vi "TDOanalysis.vi"() -> ()   [LabVIEW 2018]
uses:
  Libraries/File/Data window.ctl
  <vilib>/Analysis/4window.llb/Hanning Window (DBL).vi
  <vilib>/Analysis/4window.llb/Blackman Window (DBL).vi
  <vilib>/Analysis/baseanly.llb/Mean (DBL).vi
  <vilib>/Analysis/8numeric.llb/1D Numeric Integration.vi
  <vilib>/Analysis/4window.llb/AllCosWindow (DBL).vi
  Libraries/File/File LLB/Read any file Waveform 1ch.vi
  <vilib>/measure/matone.llb/Extract Single Tone Information 1 Chan.vi
  <vilib>/Waveform/WDTOps.llb/WDT Number of Waveform Samples DBL.vi
  <vilib>/Utility/file.llb/Write To Spreadsheet File (DBL).vi
  <vilib>/Analysis/NI_AALPro.lvlib
  <vilib>/measure/NI_MAPro.lvlib
  <vilib>/Analysis/NI_AALBase.lvlib
  <vilib>/Analysis/NI_AAL_SigProc.lvlib
panel:
  in  "Tab Control":T1(tab)
  in  "Input File":path=path "/Users/arkady/Desktop/Dropbox/local_data/rucl3-60T-Oct2018/101118/p003_101118.tdms"
  in  "Power spctr. \nAmpl. threshold":dbl=0.001 format="%.4e"
  in  "Bdot Calibration Factor":dbl=3794.0
  out "TDO Frequency vs. Field":cluster{dbl[], dbl[]}(graph)
  in  "Save Results?":bool=TRUE
  out "B dot offset":dbl=0.00015410527073910347 format="%.6f"
  in  "Data File Type":T2(ring)
  in  "Data channels (1st - Field, 2nd - TDO)":T3={"Start"=0, "Length"=10000, "Other frmt channel numbers"=[0], "TDMS Channel names"=["Field", "Vp"], "TDMS Group name"="p"}
  in  "Length for Bdot offset, s":dbl=0.009 format="%#_6p"
  in  "Input field format":enum16{"Bdot", "B"}(ring)=enum."B"
  in  "Power spctr.\nFreq. threshold":dbl=10000.0
  out "Progress":dbl(slide)=0.9998769230769231 scale=0.0..1.0
  in  "Sliding window width, s":dbl=0.0002 format="%#_6p"
  in  "Sliding window step, s":dbl=2e-05 format="%#_6p"
  in  "Frequency detection md":T4(ring)
  in  "Peak-to-peak  fit width":i32=3 min=3
  in  "Low-pass filter":T5={"Clip IIR filter ramps, in 1/Tc units"=1.0, "Two-pass & flip"=TRUE, "IIR filter specifications"={"Topology"=enum."Off", "Type"=enum."Lowpass", "Order"=1, "Lower Fc"=1e-06, "Upper Fc"=0.0, "PB Ripple"=1.0, "SB Attenuation"=60.0}} {"IIR filter specifications"."PB Ripple" format="%0.2f"; "IIR filter specifications"."Lower Fc" format="%0.2p"; "IIR filter specifications"."SB Attenuation" format="%0.2f"; "IIR filter specifications"."Upper Fc" format="%0.2p"}
  in  "Window type":enum16{"Hanning", "Box", "Blackman"}(ring)
  out "Elapsed time":dbl=1.143
  in  "Field correction":dbl=1.0
  out "Array":bool[](array[boolean])
  out "Background subtracted":cluster{"Output":dbl[], dbl[]}[](graph)
  in  "Background file":path
  out "size(s)":i32=6499
  in  "error in":errorcluster
  in  "lower limit":dbl
  in  "upper limit":dbl
  in  "# of threads":i32=4
  out "Frequency vs. time":waveform(dbl)(graph)={"t0"=timestamp(-0.010000000000000009 s since 1904-01-01), "dt"=2e-05, "Y"=array[6499 elements]}
  out "Field profile":waveform(dbl)(graph)={"t0"=timestamp(-0.010000000000000009 s since 1904-01-01), "dt"=2e-05, "Y"=array[6499 elements]}
  out "TDO Apmlitude or Pwr. vs. Field":cluster{dbl[], dbl[]}(graph)
  out "TDO Amplitude vs. Field (PWR peak)":cluster{dbl[], "Filtered X":dbl[]}(graph)
  in  "End, s":dbl=nan format="%.6f"
  in  "Start, s":dbl=nan format="%.6f"
  in  "Separate file?":bool
  in  "Input Field File (optional)":path
  # "Field  Settings"
  # "TDO Analysis Settings"
  # "Basic NHMFL TDO routine\nv. 0.5       F. F. Balakirev"
  # "OR"
  # "Background file is either an ASCII *.dat file produced by TDO earlier\nor *.fit file containing single column of polynomial fit coeficients.\n1st row in fit file is a text header, which is ingnored. Result is saved in a \n\"*diff.dat\" file in the output folder\nExample \"PDO1.fit\": \n\nFit y=A_i*x^i, starting with A_0\n3.25637E7\n2132.56863\n-12.60591\n-2.01013\n-0.04452\n-3.23119E-4"
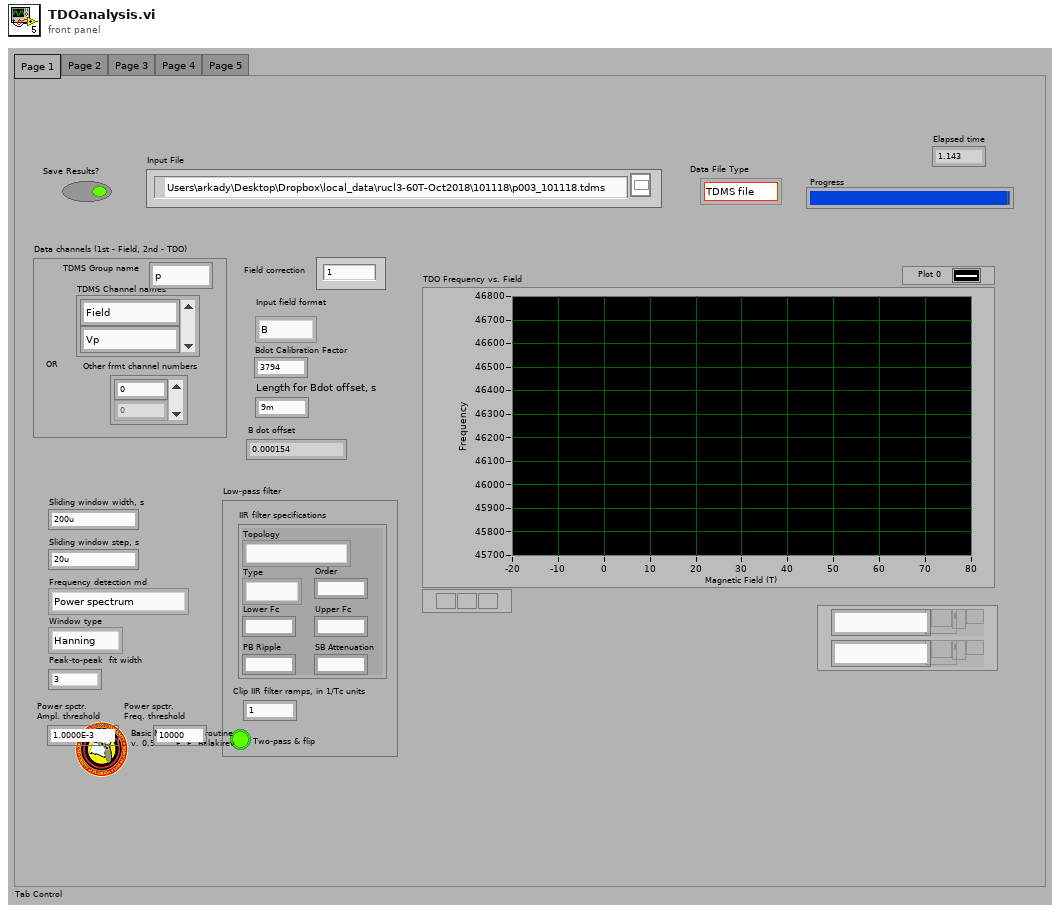
[diagram p1: front panel]
types:
  T1 = enum32{"Page 1", "Page 2", "Page 3", "Page 4", "Page 5"}
  T2 = enum16{"TDMS file", "Tektronics ISF", "BinF file", "ASCII File", "BinH File", "BinW File", "BINARY File"}
  T3 = cluster{"Start":i64, "Length":i32, "Other frmt channel numbers":i64[], "TDMS Channel names":string[], "TDMS Group name":string}
  T4 = enum16{"Power spectrum", "Tone detection", "Peak-to-peak fit"}
  T5 = cluster{"Clip IIR filter ramps, in 1/Tc units":dbl, "Two-pass & flip":bool, "IIR filter specifications":cluster{"Topology":enum16{"Off", "Butterworth", "Chebyshev", "Inverse Chebyshev", "Elliptic", "Bessel"}, "Type":enum16{"Lowpass", "Highpass", "Bandpass", "Bandstop"}, "Order":i32, "Lower Fc":dbl, "Upper Fc":dbl, "PB Ripple":dbl, "SB Attenuation":dbl}}
  T6 = typedef "Data window.ctl" = cluster{"Start":i64, "Length":i64, "Channel numbers":i64[], "Channel name":string, "Group name":string}
  T7 = enum16{"Off", "Butterworth", "Chebyshev", "Inverse Chebyshev", "Elliptic", "Bessel"}
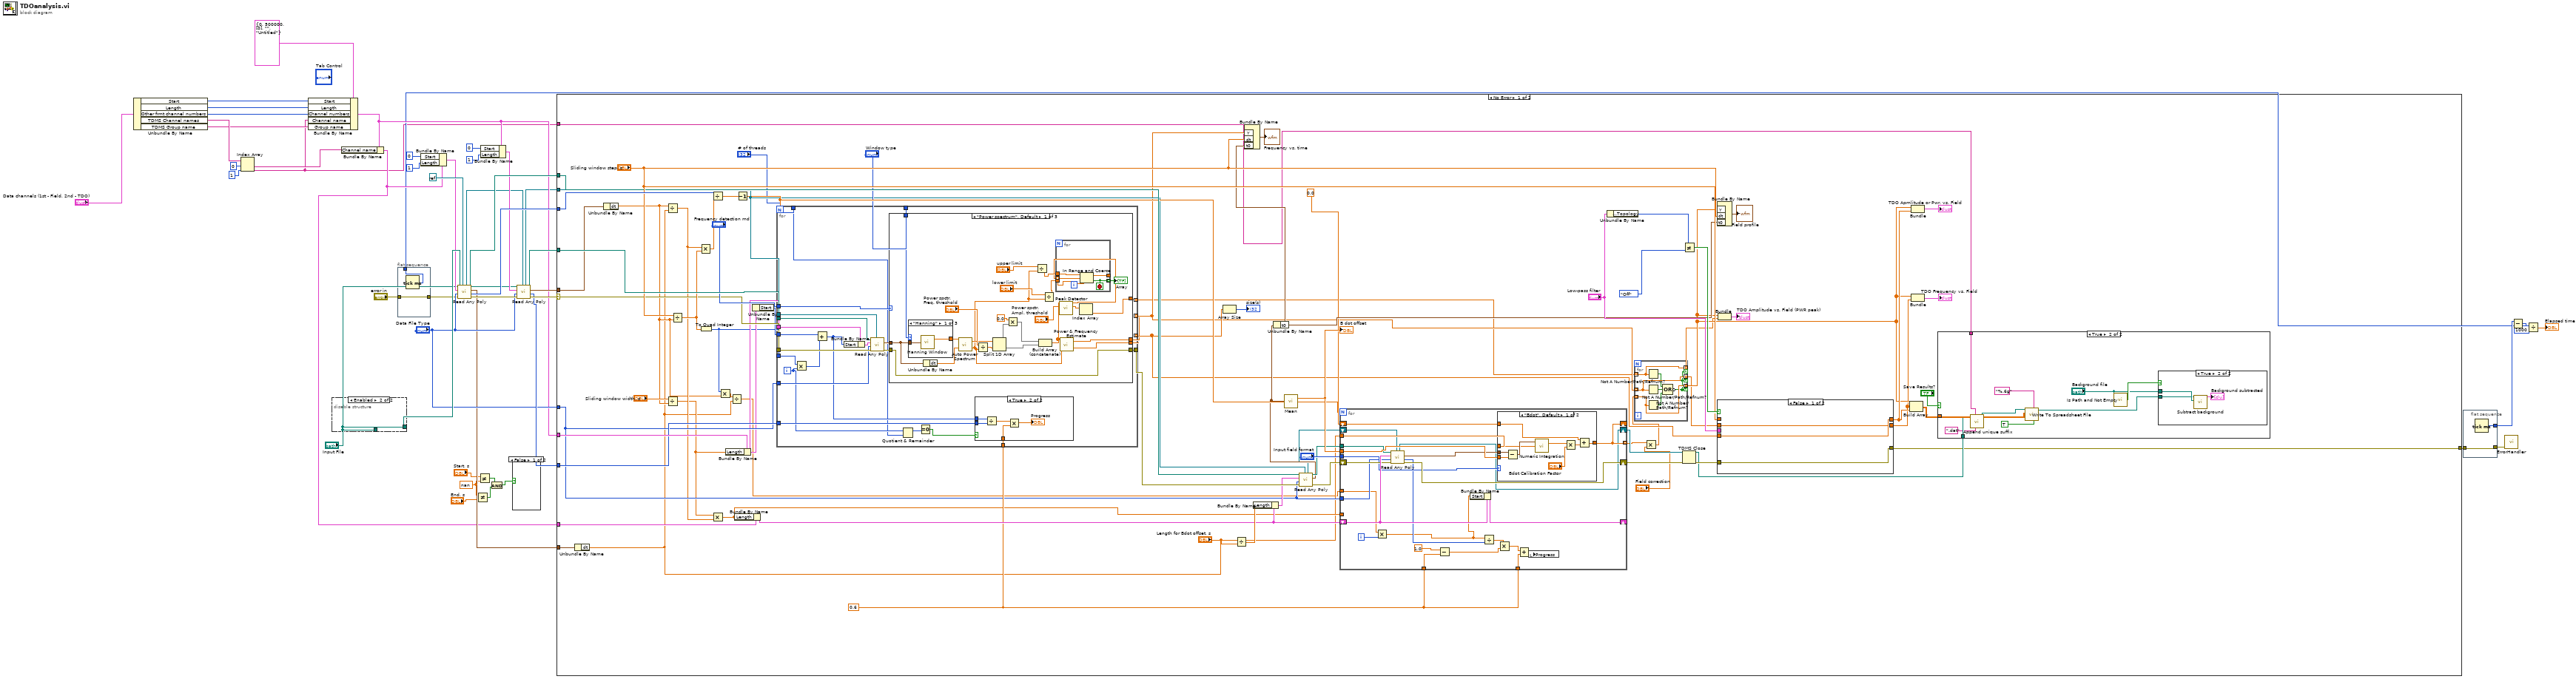
[diagram p0: block diagram]
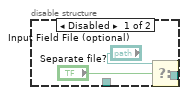
[diagram p2: hidden frame]
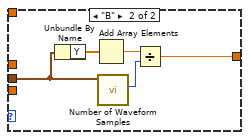
[diagram p4: hidden frame]
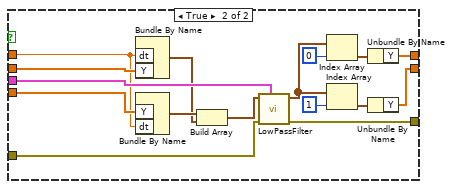
[diagram p5: hidden frame]
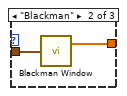
[diagram p9: hidden frame]
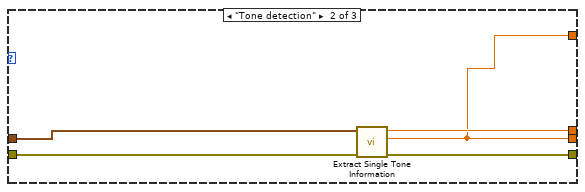
[diagram p11: hidden frame]
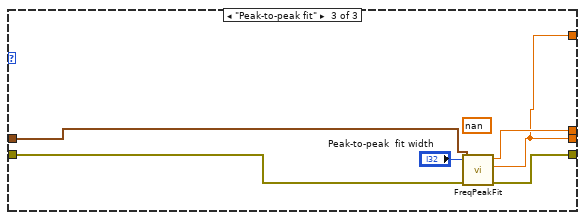
[diagram p12: hidden frame]
diagram:
  w19 = nan
  n1 = Unbundle By Name("Data channels (1st - Field, 2nd - TDO)") -> ("Start"=w30:i64, "Length"=w33:i32, "Other frmt channel numbers"=w32:i64[], "TDMS Channel names"=w35:string[], "TDMS Group name"=w31:string)
  n2 = Index Array(array=w35, index #1=0 ("index"), index #2=1 ("index")) -> (element #1=w29:string, element #2=w1:string)
  n3 = Bundle By Name(cluster=T6 {"Start"=0, "Length"=500000, "Channel numbers"=[0], "Channel name"="", "Group name"="Untitled"} ("Data window"), "Start"=w30, "Length"=w33, "Channel numbers"=w32, "Channel name"=w1, "Group name"=w31) -> (w22:T6)
  n4 = disable-structure shown="Enabled" {
    disable-tunnel: [w51 w53] -> w42
    disable-tunnel: "Input File" -> [w50 _]
    disable-tunnel: "Input File" -> [_ w53]
    frame Disabled {
      n5 = Select(t="Input Field File (optional)", s="Separate file?", f=w50) -> (s? t:f=w51:path)
    }
    frame Enabled {
    }
  }
  n6 = Bundle By Name(cluster=w22, "Channel name"=w29) -> (w25:T6)
  n7 = flat-sequence {
    tunnel: "error in" -> [w55]
    tunnel: [w55] -> w13
    tunnel: [w54] -> w9
    frame #0 {
      n8 = Tick Count (ms)() -> (millisecond timer value=w54:u32)
    }
  }
  n9 = Bundle By Name(cluster=w25, "Start"=0, "Length"=1) -> (w26:T6)
  n10 = call-poly "Read Any Poly.vi"("tdms file in"=refnum<k0> refnum, "error in"=w13, "Data File Type"="Data File Type", "Data window"=w26, "Input file path"=w42) -> ("error out"=w47:errorcluster, "1st channel length"=w39:u64, "Data out"=w28:waveform(dbl), "Actual input file path"=w41:path, "tdms file out"=w3:refnum<k34>)  [unwired: 1 in, 1 out]
  n11 = Not Equal?(x=w19, y="End, s") -> (x != y?=w16:bool)
  n12 = Not Equal?(x="Start, s", y=w19) -> (x != y?=w17:bool)
  n13 = Bundle By Name(cluster=w22, "Start"=0, "Length"=1) -> (w21:T6)
  n14 = And(x=w17, y=w16) -> (x .and. y?=w15:bool)
  n15 = case shown="False" w15 {
    frame False {
    }
    frame True {
    }
  }
  n16 = call-poly "Read Any Poly.vi"("tdms file in"=w3, "error in"=w47, "Data File Type"="Data File Type", "Data window"=w21, "Input file path"="Input File") -> ("error out"=w43:errorcluster, "1st channel length"=w38:u64, "Data out"=w44:waveform(dbl), "Actual input file path"=w46:path, "tdms file out"=w5:refnum<k34>)  [unwired: 1 in, 1 out]
  n17 = case shown="No Error" w43 {
    selector: w43 -> [w82 w282]
    tunnel: w28 -> [w91 _]
    tunnel: w22 -> [w121 _]
    tunnel: w46 -> [w120 _]
    tunnel: w44 -> [w90 _]
    tunnel: "Data File Type" -> [w83 _]
    tunnel: w39 -> [w116 _]
    tunnel: [w69 w282] -> w12
    tunnel: w41 -> [w106 _]
    tunnel: w38 -> [w93 _]
    tunnel: w25 -> [w89 _]
    tunnel: w5 -> [w68 _]
    tunnel: w1 -> [w59 _]
    frame No Error {
      w92 = 0.6 ("y")
      n18 = Unbundle By Name(w91) -> ("dt"=w71:dbl)
      n19 = Unbundle By Name(w90) -> ("dt"=w73:dbl)
      n20 = Divide(x=w73, y=w71) -> (x/y=w81:dbl)
      n21 = Divide(x="Sliding window width, s", y=w73) -> (x/y=w75:dbl)
      n22 = Divide(x="Sliding window step, s", y=w73) -> (x/y=w118:dbl)
      n23 = Multiply(x=w81, y=w118) -> (x*y=w101:dbl)
      n24 = To Quad Integer(1:w118) -> (0:w74:i64)
      n25 = Divide(x=w116, y=w101) -> (x/y=w128:dbl)
      n26 = Multiply(x=w75, y=w81) -> (x*y=w76:dbl)
      n27 = Multiply(x=w74, y=w73) -> (x*y=w72:dbl)
      n28 = Bundle By Name(cluster=w121, "Length"=w75) -> (w80:T6)
      n29 = Divide(x=w72, y=w71) -> (x/y=w70:dbl)
      n30 = Bundle By Name(cluster=w89, "Length"=w76) -> (w102:T6)
      n31 = Decrement(x=w128) -> (x-1=w94:dbl)
      n32 = Unbundle By Name(w80) -> ("Start"=w79:i64)
      n33 = for {
        N: w94 -> [_]
        tunnel: [w225] -> w64 mode=indexing
        tunnel: [w230] -> w65 mode=indexing
        tunnel: [w229] -> w63 mode=indexing
        tunnel: w83 -> [w226]
        tunnel: w120 -> [w227]
        tunnel: w74 -> [w218]
        tunnel: "Frequency detection md" -> [w224]
        tunnel: w93 -> [w223]
        tunnel: w92 -> [w220]
        tunnel: w80 -> [w217]
        tunnel: w79 -> [w216]
        tunnel: w82 -> [w228]
        tunnel: [w222] -> w96
        tunnel: "Window type" -> [w214]
        tunnel: w68 -> [w208]
        tunnel: "# of threads" -> [w207]
        i -> [w211]
        n34 = Multiply(x=w218, y=w211) -> (x*y=w212:i64)
        n35 = Add(x=w216, y=w212) -> (x+y=w213:i64)
        n36 = Bundle By Name(cluster=w217, "Start"=w213) -> (w215:T6)
        n37 = call-poly "Read Any Poly.vi"("tdms file in"=w208, "error in"=w228, "Data File Type"=w226, "Data window"=w215, "Input file path"=w227) -> ("error out"=w221:errorcluster, "Data out"=w219:waveform(dbl))  [unwired: 1 in, 4 out]
        n38 = case shown="\"Power spectrum\", Default" w224 {
          tunnel: [w259 w271 w276] -> w230
          tunnel: [w240 w271 w276] -> w229
          tunnel: w219 -> [w258 w274 w281]
          tunnel: [w247 w275 w280] -> w225
          tunnel: w221 -> [w249 w273 w278]
          tunnel: [w249 w272 w277] -> w222
          tunnel: w214 -> [w248 _ _]
          frame "Power spectrum", Default {
            n39 = case shown="\"Hanning\"" w248 {
              tunnel: [w267 w269 w270] -> w260
              tunnel: w258 -> [w266 w268 w270]
              frame "Hanning" {
                n40 = call-poly <vilib>:"Hanning Window.vi"("X"=w266) -> ("Windowed X"=w267:dbl[])  [unwired: 1 out]
              }
              frame "Blackman" {
                n41 = call-poly <vilib>:"Blackman Window.vi"("X"=w268) -> ("Windowed X"=w269:dbl[])  [unwired: 1 out]
              }
              frame "Box" {
              }
            }
            n42 = Unbundle By Name(w258) -> ("dt"=w257:dbl)
            n43 = call <vilib>:"Auto Power Spectrum.vi"("dt"=w257, "Signal (V)"=w260) -> ("df"=w244:dbl, "Power Spectrum (V^2 rms)"=w255:dbl[])
            n44 = Divide(x="Power spctr.\nFreq. threshold", y=w244) -> (x/y=w254:dbl)
            n45 = Split 1D Array(array=w255, index=w254) -> (first subarray=w251:dbl[], second subarray=w253:dbl[])
            n46 = Multiply(x=0.0 ("element"), y=w251) -> (x*y=w250:dbl[])
            n47 = Divide(x="upper limit", y=w244) -> (x/y=w242:dbl)
            n48 = Build Array (concatenate)(w250, w253) -> (w239:dbl[])
            n49 = Divide(x="lower limit", y=w244) -> (x/y=w245:dbl)
            n50 = call <vilib>:"Peak Detector.vi"("threshold"="Power spctr. \nAmpl. threshold", "X"=w239) -> ("Amplitudes"=w236:dbl[], "Locations"=w237:dbl[])  [unwired: 5 in, 3 out]
            n51 = for {
              tunnel: w237 -> [w265] mode=indexing
              tunnel: w242 -> [w264]
              tunnel: w245 -> [w263]
              tunnel: [w262] -> _
              tunnel: [w261] -> w241 mode=indexing
              stop <- w261 stop-if-true
              n52 = In Range and Coerce(upper limit=w264, x=w265, lower limit=w263) -> (coerced(x)=w262:dbl, In Range?=w261:bool)
            }
            "Array" <- w241
            n53 = call <vilib>:"Power & Frequency Estimate.vi"("df"=w244, "Power Spectrum (V^2 rms)"=w239) -> ("est power peak"=w259:dbl, "est frequency peak"=w247:dbl)  [unwired: 3 in, 1 out]
            n54 = Index Array(array=w236) -> (element=w240:dbl)  [unwired: 1 in]
          }
          frame "Tone detection" {
            n55 = call-poly <vilib>:"Extract Single Tone Information.vi"("error in (no error)"=w273, "time signal in"=w274) -> ("error out"=w272:errorcluster, "detected amplitude"=w271:dbl, "detected frequency"=w275:dbl)  [unwired: 2 in, 5 out]
          }
          frame "Peak-to-peak fit" {
            (unwired) nan
            n56 = call "FreqPeakFit.vi"("error in (no error)"=w278, "Peak fit width"="Peak-to-peak  fit width", "Waveform"=w281) -> ("error out"=w277:errorcluster, "Amplitude"=w276:dbl, "PeakFreqOut"=w280:dbl)  [unwired: 4 out]
          }
        }
        n57 = Quotient & Remainder(x=w211, y=w207) -> (x-y*floor(x/y)=w210:i32)  [unwired: 1 out]
        n58 = Equal To 0?(x=w210) -> (x = 0?=w209:bool)
        n59 = case shown="True" w209 {
          tunnel: w223 -> [_ w235]
          tunnel: w220 -> [_ w232]
          tunnel: w213 -> [_ w231]
          frame False {
          }
          frame True {
            n60 = Divide(x=w231, y=w235) -> (x/y=w234:dbl)
            n61 = Multiply(x=w234, y=w232) -> (x*y=→"Progress":dbl)
          }
        }
      }
      n62 = Array Size(array=w65) -> (size(s)=→"size(s)":i32)
      n63 = Divide(x="Length for Bdot offset, s", y=w71) -> (x/y=w104:dbl)
      n64 = Bundle By Name(cluster=w102, "Length"=w104) -> (w88:T6)
      n65 = call-poly "Read Any Poly.vi"("tdms file in"=w68, "error in"=w96, "Data File Type"=w83, "Data window"=w88, "Input file path"=w106) -> ("error out"=w95:errorcluster, "Data out"=w87:waveform(dbl), "Actual input file path"=w97:path, "tdms file out"=w86:refnum<k34>)  [unwired: 1 in, 2 out]
      n66 = Unbundle By Name(w87) -> ("t0"=w107:timestamp)
      n67 = Bundle By Name("Y"=w64, "dt"="Sliding window step, s", "t0"=w107) -> (→"Frequency vs. time":waveform(dbl))  [unwired: 1 out]
      n68 = call-poly <vilib>:"Mean.vi"("X"=w87) -> ("mean"=w99:dbl)  [unwired: 1 out]
      "B dot offset" <- w99
      n69 = for {
        N: w94 -> [_]
        shift-right: [w157] -> w103
        shift-left: w95 -> [w158]
        shift-right: [w160] -> _
        shift-left: w102 -> [w159]
        tunnel: w70 -> [w137]
        tunnel: "Input field format" -> [w156]
        tunnel: w99 -> [w155]
        shift-right: [w154] -> _
        shift-left: 0.0 -> [w153]
        tunnel: [w154] -> w58 mode=indexing
        tunnel: w71 -> [w152]
        tunnel: w97 -> [w151]
        tunnel: w92 -> [w147]
        tunnel: w92 -> [w143]
        shift-right: [w140] -> w84
        shift-left: w86 -> [w141]
        tunnel: w83 -> [w139]
        tunnel: w76 -> [_]
        i -> [w138]
        n70 = Multiply(x=w137, y=w138) -> (x*y=w136:dbl)
        n71 = call-poly "Read Any Poly.vi"("tdms file in"=w141, "error in"=w158, "Data File Type"=w139, "Data window"=w159, "Input file path"=w151) -> ("error out"=w157:errorcluster, "1st channel length"=w149:u64, "Data out"=w142:waveform(dbl), "tdms file out"=w140:refnum<k34>)  [unwired: 1 in, 2 out]
        n72 = Subtract(x=1.0, y=w147) -> (x-y=w146:dbl)
        n73 = Bundle By Name(cluster=w159, "Start"=w136) -> (w160:T6)
        n74 = Divide(x=w136, y=w149) -> (x/y=w150:dbl)
        n75 = case shown="\"Bdot\", Default" w156 {
          tunnel: w153 -> [w169 _]
          tunnel: [w167 w171] -> w154
          tunnel: w155 -> [w165 _]
          tunnel: w152 -> [w163 _]
          tunnel: w142 -> [w162 w170]
          frame "Bdot", Default {
            n76 = Subtract(x=w162, y=w165) -> (x-y=w166:waveform(dbl))
            n77 = call-poly <vilib>:"Numeric Integration.vi"("dt"=w163, "Input Array"=w166) -> ("result"=w164:dbl)  [unwired: 1 in, 1 out]
            n78 = Multiply(x=w164, y="Bdot Calibration Factor") -> (x*y=w168:dbl)
            n79 = Add(x=w169, y=w168) -> (x+y=w167:dbl)
          }
          frame "B" {
            n80 = Unbundle By Name(w170) -> ("Y"=w174:dbl[])
            n81 = Add Array Elements(numeric array=w174) -> (sum=w172:dbl)
            n82 = call-poly <vilib>:"Number of Waveform Samples.vi"("waveform in"=w170) -> ("number of samples"=w173:i32)  [unwired: 1 in, 9 out]
            n83 = Divide(x=w172, y=w173) -> (x/y=w171:dbl)
          }
        }
        n84 = Multiply(x=w150, y=w146) -> (x*y=w144:dbl)
        n85 = Add(x=w144, y=w143) -> (x+y=w145:dbl)
        n86 = local write "Progress"(w145) -> ()
      }
      n87 = Unbundle By Name("Low-pass filter") -> ("IIR filter specifications.Topology"=w114:T7)
      n88 = Multiply(x=w58, y="Field correction") -> (x*y=w56:dbl[])
      n89 = for {
        tunnel: w64 -> [w134] mode=indexing
        tunnel: w56 -> [w133] mode=indexing
        tunnel: w63 -> [w135] mode=indexing
        tunnel: [w135] -> w60 mode=indexing if=w129
        tunnel: [w134] -> w61 mode=indexing if=w129
        tunnel: [w133] -> w67 mode=indexing if=w129
        n90 = Not A Number/Path/Refnum?(number/path/refnum=w135) -> (NaN/Path/Refnum?=w132:bool)
        n91 = Not A Number/Path/Refnum?(number/path/refnum=w134) -> (NaN/Path/Refnum?=w131:bool)
        n92 = Not A Number/Path/Refnum?(number/path/refnum=w133) -> (NaN/Path/Refnum?=w130:bool)
        n93 = Compound Arithmetic op=OR(w132, w131, w130) -> (invert w129:bool)
      }
      n94 = TDMS Close(8:w103, 11:w84) -> (0:w85:errorcluster, 3:w77:path)
      n95 = Not Equal?(x=w114, y=T7."Off" ("IIR filter specifications.Topology")) -> (x != y?=w113:bool)
      n96 = Bundle By Name("Y"=w67, "dt"="Sliding window step, s", "t0"=w107) -> (→"Field profile":waveform(dbl))  [unwired: 1 out]
      n97 = case shown="False" w113 {
        tunnel: w85 -> [w177 w193]
        tunnel: [w177 w192] -> w69
        tunnel: "Low-pass filter" -> [_ w191]
        tunnel: w65 -> [w176 w189]
        tunnel: w61 -> [w175 w190]
        tunnel: "Sliding window step, s" -> [_ w178]
        tunnel: [w175 w180] -> w62
        tunnel: [w176 w179] -> w111
        frame False {
        }
        frame True {
          n98 = Bundle By Name("dt"=w178, "Y"=w190) -> (w187:waveform(dbl))  [unwired: 1 out]
          n99 = Bundle By Name("Y"=w189, "dt"=w178) -> (w188:waveform(dbl))  [unwired: 1 out]
          n100 = Build Array(w188, w187) -> (w186:waveform(dbl)[])
          n101 = call "LowPassFilter.vi"("Low-pass filter"=w191, "error in (no error)"=w193, "signal(s) in"=w186) -> ("error out"=w192:errorcluster, "signal(s) out"=w185:waveform(dbl)[])  [unwired: 2 in, 5 out]
          n102 = Index Array(array=w185, index=0) -> (element=w182:waveform(dbl))
          n103 = Index Array(array=w185, index=1) -> (element=w181:waveform(dbl))
          n104 = Unbundle By Name(w182) -> ("Y"=w179:dbl[])
          n105 = Unbundle By Name(w181) -> ("Y"=w180:dbl[])
        }
      }
      n106 = Bundle(w67, w60) -> (→"TDO Amplitude vs. Field (PWR peak)":cluster{dbl[], dbl[]})  [unwired: 1 out]
      n107 = Build Array(w67, w62, w111) -> (w126:dbl[][])
      n108 = Bundle(w67, "Y"=w111) -> (→"TDO Apmlitude or Pwr. vs. Field":cluster{dbl[], "Y":dbl[]})  [unwired: 1 out]
      n109 = Bundle(w67, "Y"=w62) -> (→"TDO Frequency vs. Field":cluster{dbl[], "Y":dbl[]})  [unwired: 1 out]
      n110 = case shown="True" "Save Results?" {
        tunnel: w126 -> [_ w203]
        tunnel: w77 -> [_ w200]
        tunnel: w59 -> [_ w197]
        frame False {
        }
        frame True {
          n111 = call "Append unique suffix.vi"("Extention"=".dat", "Suffix"=w197, "Path"=w200) -> ("Path out"=w199:path)  [unwired: 7 in, 1 out]
          n112 = call-poly <vilib>:"Write To Spreadsheet File.vi"("transpose? (no:F)"=TRUE, "format (%.3f)"="%.6g", "2D data"=w203, "file path (dialog if empty)"=w199) -> ("new file path (Not A Path if cancelled)"=w194:path)  [unwired: 2 in, 2 out]
          n113 = call <vilib>:"Is Path and Not Empty.vi"("path"="Background file") -> ("Is Path and Not Empty?"=w196:bool)  [unwired: 4 in]
          n114 = case shown="True" w196 {
            tunnel: "Background file" -> [_ w206]
            tunnel: w194 -> [_ w205]
            frame False {
            }
            frame True {
              n115 = call "Subtract background.vi"("Background"=w206, "Data"=w205) -> ("XY Graph"=→"Background subtracted":cluster{"Output":dbl[], dbl[]}[])  [unwired: 9 in]
            }
          }
        }
      }
    }
    frame Error {
    }
  }
  n116 = flat-sequence {
    tunnel: w12 -> [w284]
    tunnel: [w284] -> w11
    tunnel: [w283] -> w10
    frame #0 {
      n117 = Tick Count (ms)() -> (millisecond timer value=w283:u32)
    }
  }
  n118 = call "ErrorHandler.vi"("error in (no error)"=w11) -> ()  [unwired: 1 in, 10 out]
  n119 = Subtract(x=w10, y=w9) -> (x-y=w8:u32)
  n120 = Divide(x=w8, y=u32 1000) -> (x/y=→"Elapsed time":dbl)
